vi "Insert Specifical Controls to [4,4] Array.vi"(7 "controls references":refnum<vi>[](array[refnum]), 8 "error in":errorcluster {"code" format="%.0x"}, 9 "2-D controls references":refnum<vi>[][](array[refnum]), 10 "indicators":refnum<vi>[](array[refnum]), 11 "controls":refnum<vi>[](array[refnum])) -> (0 "error out":errorcluster {"code" format="%.0x"}, 1 "2-D controls references out":refnum<vi>[][](array[refnum]), 2 "indicators out":refnum<vi>[](array[refnum]), 3 "controls out":refnum<vi>[](array[refnum]), 4 "controls references out":refnum<vi>[](array[refnum]))   [LabVIEW 2018, in "NISAST VI Scripting.lvlib" / "VI.lvlib" / "Front Panel.lvlib"]
uses:
  Front Panel.lvlib
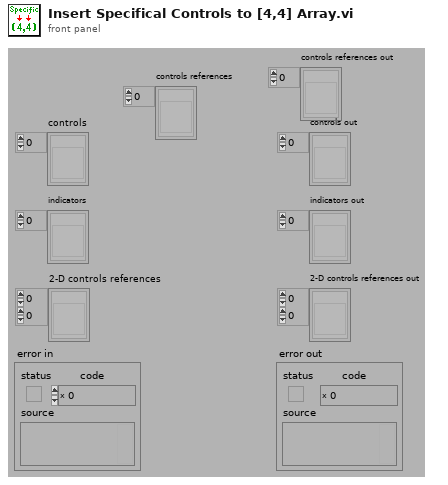
[diagram p1: front panel]
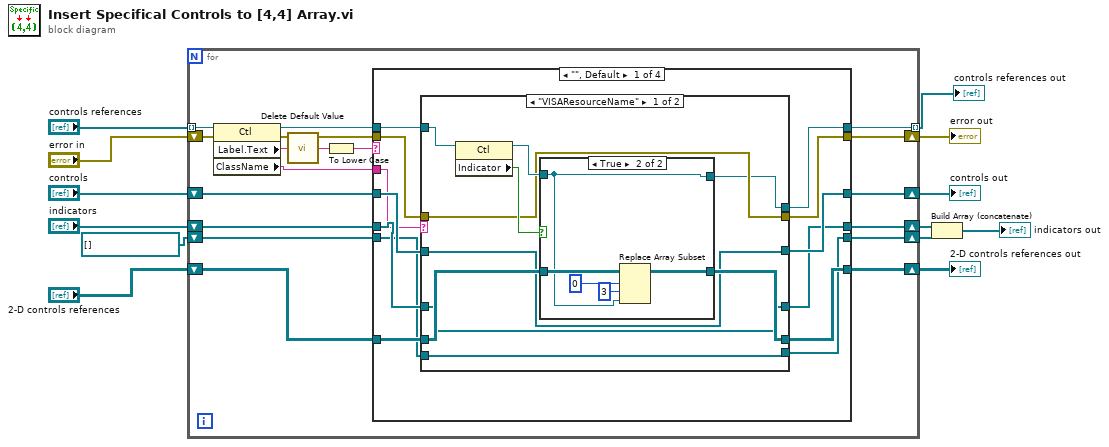
[diagram p0: block diagram]
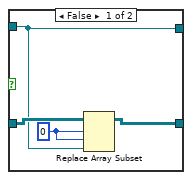
[diagram p2: hidden frame]
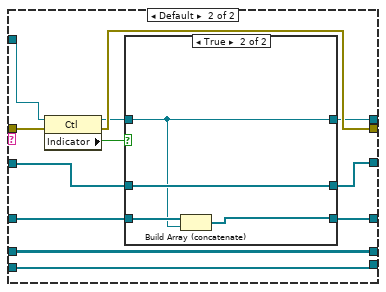
[diagram p3: hidden frame]
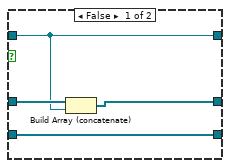
[diagram p4: hidden frame]
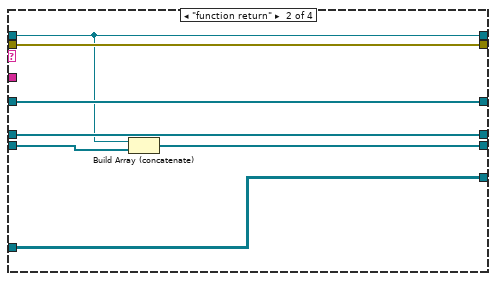
[diagram p5: hidden frame]
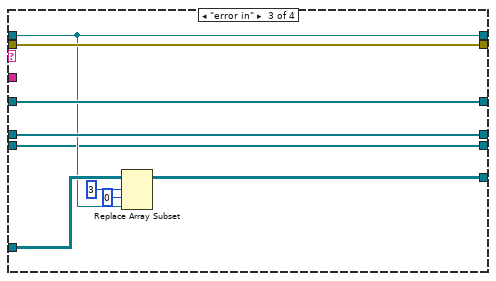
[diagram p6: hidden frame]
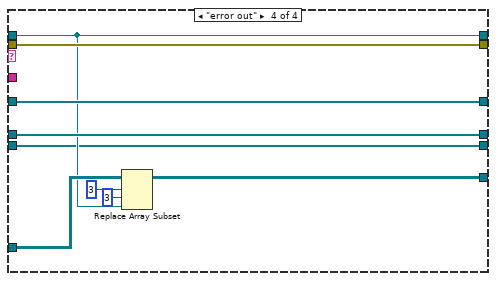
[diagram p7: hidden frame]
diagram:
  n1 = for {
    tunnel: "controls references" -> [w31] mode=indexing
    shift-right: [w28] -> w8
    shift-left: "2-D controls references" -> [w30]
    shift-right: [w27] -> w9
    shift-left: "controls" -> [w26]
    shift-right: [w24] -> w4
    shift-left: "indicators" -> [w25]
    shift-right: [w21] -> w6
    shift-left: "error in" -> [w22]
    tunnel: [w17] -> w5 mode=indexing
    shift-right: [w16] -> w2
    shift-left: refnum<vi>[] [] -> [w15]
    n2 = property class="Ctl"(reference=w31, error in=w22) -> (reference out=w29:refnum<vi>, error out=w23:errorcluster, "Label.Text"=w19:string, "ClassName"=w14:string)
    n3 = call "Delete Default Value.vi"("label or caption"=w19) -> ("naked label or caption"=w18:string)  [unwired: 4 out]
    n4 = To Lower Case(string=w18) -> (all lower case string=w20:string)
    n5 = case shown="\"\", Default" w20 {
      tunnel: w30 -> [w35 w90 w99 w108]
      tunnel: w29 -> [w44 w84 w92 w101]
      tunnel: [w36 w90 w96 w105] -> w28
      tunnel: [w43 w89 w95 w104] -> w27
      tunnel: w26 -> [w42 w89 w95 w104]
      tunnel: w25 -> [w41 w87 w94 w103]
      tunnel: [w40 w87 w94 w103] -> w24
      tunnel: w23 -> [w39 w88 w93 w102]
      tunnel: [w38 w88 w93 w102] -> w21
      tunnel: [w37 w84 w92 w101] -> w17
      tunnel: [w33 w85 w91 w100] -> w16
      tunnel: w15 -> [w34 w86 w91 w100]
      tunnel: w14 -> [w32 _ _ _]
      frame "", Default {
        n6 = case shown="\"VISAResourceName\"" w32 {
          tunnel: w44 -> [w54 w75]
          tunnel: [w46 w74] -> w43
          tunnel: w42 -> [w46 w73]
          tunnel: w41 -> [w45 w72]
          tunnel: [w45 w71] -> w40
          tunnel: w39 -> [w48 w70]
          tunnel: [w48 w69] -> w38
          tunnel: [w47 w68] -> w37
          tunnel: [w50 w65] -> w36
          tunnel: w35 -> [w51 w65]
          tunnel: [w49 w64] -> w33
          tunnel: w34 -> [w49 w64]
          frame "VISAResourceName" {
            n7 = property class="Ctl"(reference=w54) -> (reference out=w52:refnum<vi>, "Indicator"=w53:bool)  [unwired: 1 in, 1 out]
            n8 = case shown="True" w53 {
              tunnel: w52 -> [w55 w59]
              tunnel: w51 -> [w58 w63]
              tunnel: [w57 w60] -> w50
              tunnel: [w55 w59] -> w47
              frame False {
                w56 = 0 ("index (row)")
                n9 = Replace Array Subset(array=w58, new element=w55, index (row)=w56, index (col)=w56) -> (w57:refnum<vi>[][])
              }
              frame True {
                n10 = Replace Array Subset(array=w63, new element=w59, index (row)=0, index (col)=3 ("disabled index (col)")) -> (w60:refnum<vi>[][])
              }
            }
          }
          frame Default {
            n11 = property class="Ctl"(reference=w75, error in=w70) -> (reference out=w66:refnum<vi>, error out=w69:errorcluster, "Indicator"=w67:bool)
            n12 = case shown="True" w67 {
              tunnel: w66 -> [w76 w80]
              tunnel: [w79 w81] -> w74
              tunnel: w73 -> [w78 w81]
              tunnel: [w77 w83] -> w71
              tunnel: w72 -> [w77 w82]
              tunnel: [w76 w80] -> w68
              frame False {
                n13 = Build Array (concatenate)(w78, w76) -> (w79:refnum<vi>[])
              }
              frame True {
                n14 = Build Array (concatenate)(w82, w80) -> (w83:refnum<vi>[])
              }
            }
          }
        }
      }
      frame "function return" {
        n15 = Build Array (concatenate)(w84, w86) -> (w85:refnum<vi>[])
      }
      frame "error in" {
        n16 = Replace Array Subset(array=w99, new element=w92, index (row)=3 ("Disabled Index (row)"), index (col)=0 ("Disabled Index (col)")) -> (w96:refnum<vi>[][])
      }
      frame "error out" {
        n17 = Replace Array Subset(array=w108, new element=w101, index (row)=3 ("Disabled Index (row)"), index (col)=3 ("Disabled Index (col)")) -> (w105:refnum<vi>[][])
      }
    }
  }
  "controls out" <- w9
  "2-D controls references out" <- w8
  "error out" <- w6
  "controls references out" <- w5
  n18 = Build Array (concatenate)(w4, w2) -> (→"indicators out":refnum<vi>[])
